vi "MockFAILC2.vi"(11 "MockFAILC2Settings":T1={"ModbusTxDataFIFO"="ModbusSubnetBTxDataFIFO", "Code17Memory"="MockFAILC2Code17", "BufferUpdateFIFO"="MockFAILC2Command", "ModbusRxDataFIFO"="ModbusSubnetBRxDataFIFO", "Code18Memory"="MockFAILC2Code18", "Code65Memory"="MockFAILC2Code65", "Code66Memory"="MockFAILC2Code66", "Code67Memory"="MockFAILC2Code67", "Code72Memory"="MockFAILC2Code72", "Code80Memory"="MockFAILC2Code80", "Code110Memory"="MockFAILC2Code110", "CRCDataFIFO"="MockFAILC2CRCDataFIFO", "CRCCalculateFIFO"="MockFAILC2CRCCalculateFIFO", "CRCFIFO"="MockFAILC2CRCFIFO"}) -> ()   [LabVIEW 2016]
uses:
  Common_FPGA_Modbus/DataTypes/ModbusCRCSettings.ctl
  DataTypes/MockFAILC2Settings.ctl
  Common_FPGA_Modbus/FPGAModbus.lvlib
  FPGAMockFAILC.lvlib
panel:
  in  "ModbusCRCSettings":T2={"DataFIFO"="MockFAILC2CRCDataFIFO", "CalculateFIFO"="MockFAILC2CRCCalculateFIFO", "OutputFIFO"="MockFAILC2CRCFIFO"}
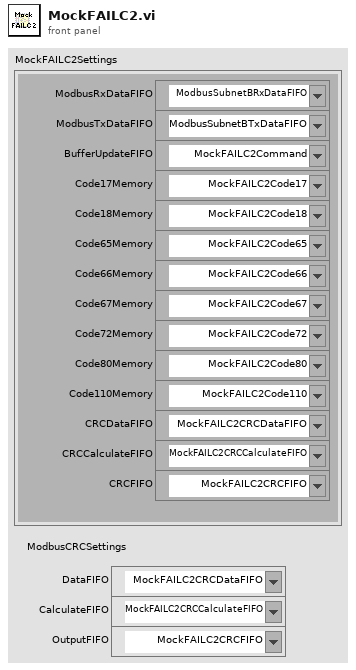
[diagram p1: front panel]
types:
  T1 = typedef "FPGAMockFAILC.lvlib/MockFAILC2Settings.ctl" = cluster{"ModbusTxDataFIFO":refnum<k21>, "Code17Memory":refnum<k21>, "BufferUpdateFIFO":refnum<k21>, "ModbusRxDataFIFO":refnum<k21>, "Code18Memory":refnum<k21>, "Code65Memory":refnum<k21>, "Code66Memory":refnum<k21>, "Code67Memory":refnum<k21>, "Code72Memory":refnum<k21>, "Code80Memory":refnum<k21>, "Code110Memory":refnum<k21>, "CRCDataFIFO":refnum<k21>, "CRCCalculateFIFO":refnum<k21>, "CRCFIFO":refnum<k21>}
  T2 = typedef "FPGAModbus.lvlib/ModbusCRCSettings.ctl" = cluster{"DataFIFO":refnum<k21>, "CalculateFIFO":refnum<k21>, "OutputFIFO":refnum<k21>}
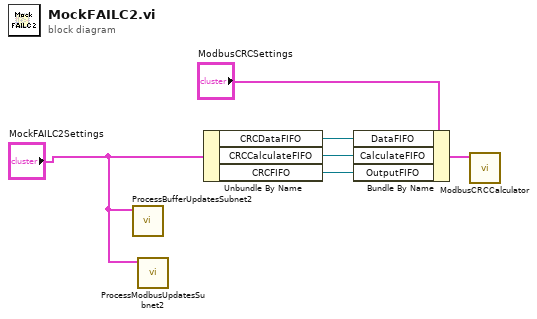
[diagram p0: block diagram]
diagram:
  n1 = call "ProcessBufferUpdatesSubnet2.vi"("MockFAILC2Settings"="MockFAILC2Settings") -> ()  [unwired: 11 in]
  n2 = call "ProcessModbusUpdatesSubnet2.vi"("MockFAILC2Settings"="MockFAILC2Settings") -> ()  [unwired: 11 in]
  n3 = Unbundle By Name("MockFAILC2Settings") -> ("CRCDataFIFO"=w3:refnum<k21>, "CRCCalculateFIFO"=w4:refnum<k21>, "CRCFIFO"=w5:refnum<k21>)
  n4 = Bundle By Name(cluster="ModbusCRCSettings", "DataFIFO"=w3, "CalculateFIFO"=w4, "OutputFIFO"=w5) -> (w6:T2)
  n5 = call "ModbusCRCCalculator.vi"("ModbusCRCSettings"=w6) -> ()  [unwired: 11 in]
